vi "GetSubVI Paths.vi"(11 "Dependency Paths":path[](array[path])) -> (2 "DriverVIs":path[](array[path]), 3 "ActualDependencies[]":path[](array[path]))   [LabVIEW 2021, in "Converter.lvlib"]
uses:
  Converter.lvlib
  Converter Reusables/Converter Reusables.lvlib
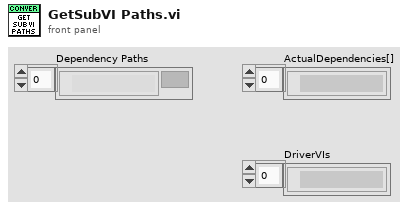
[diagram p1: front panel]
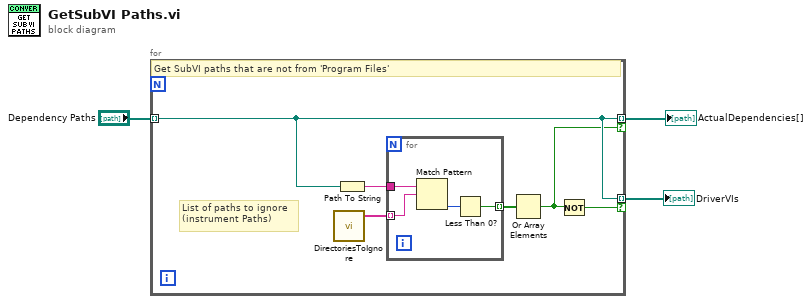
[diagram p0: block diagram]
diagram:
  n1 = for {
    tunnel: "Dependency Paths" -> [w8] mode=indexing
    tunnel: [w8] -> w3 mode=indexing if=w4
    tunnel: [w8] -> w1 mode=indexing if=w6
    # "List of paths to ignore\n(instrument Paths)"
    # "Get SubVI paths that are not from 'Program Files'"
    n2 = call "DirectoriesToIgnore.vi"() -> ("IgnoredDirectories[]"=w5:string[])  [unwired: 5 in]
    n3 = Path To String(path=w8) -> (string=w9:string)
    n4 = for {
      tunnel: w9 -> [w13]
      tunnel: [w10] -> w7 mode=indexing
      tunnel: w5 -> [w11] mode=indexing
      n5 = Match Pattern(string=w13, regular expression=w11) -> (offset past match=w12:i32)  [unwired: 1 in, 3 out]
      n6 = Less Than 0?(x=w12) -> (x < 0?=w10:bool)
    }
    n7 = Or Array Elements(Boolean array=w7) -> (logical OR=w4:bool)
    n8 = Not(x=w4) -> (.not. x?=w6:bool)
  }
  "ActualDependencies[]" <- w3
  "DriverVIs" <- w1
